vi "Helper SubVI - Plot Integer Histogram.vi"(9 "2D integer signal":i32[][](array[numeric])) -> (1 "histogram":cluster{"x":dbl[], "Histogram":i32[]})   [LabVIEW 2023]
doc: "Calculates the 2D IWT histrogram."
uses:
  <vilib>/Analysis/NI_AALPro.lvlib
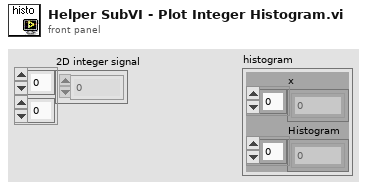
[diagram p1: front panel]
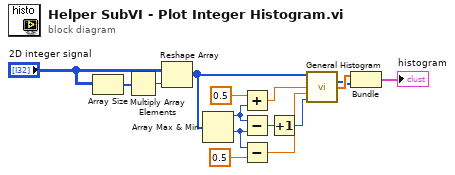
[diagram p0: block diagram]
diagram:
  n1 = Array Size(array="2D integer signal") -> (size(s)=w1:i32[])
  n2 = Multiply Array Elements(1:w1) -> (0:w2:i32)
  n3 = Reshape Array("2D integer signal", w2) -> (w3:i32[])
  n4 = Array Max & Min(array=w3) -> (max value=w4:i32, min value=w6:i32)  [unwired: 2 out]
  n5 = Add(x=0.5, y=w4) -> (x+y=w9:dbl)
  n6 = Subtract(x=w4, y=w6) -> (x-y=w10:i32)
  n7 = Subtract(x=w6, y=0.5 ("x")) -> (x-y=w8:dbl)
  n8 = Increment(x=w10) -> (x+1=w11:i32)
  n9 = call <vilib>:"General Histogram.vi"("X"=w3, "max"=w9, "min"=w8, "# bins"=w11) -> ("Histogram"=w12:i32[], "Axis"=w13:dbl[])  [unwired: 2 in, 8 out]
  n10 = Bundle("Axis"=w13, "Histogram"=w12) -> (→"histogram":cluster{"Axis":dbl[], "Histogram":i32[]})  [unwired: 1 out]
